vi "PH_Tektronix_7000.set Graph GUI Element.vi"(0 "i ref in":refnum<vi>, 5 "error in (no error)":errorcluster) -> (14 "i ref out":refnum<vi>, 19 "error out":errorcluster)   [LabVIEW 2014, in "PH_Tektronix_7000.lvlib"]
doc: "This sets the Graph GUI Element."
uses:
  PH_Tektronix_7000.lvlib
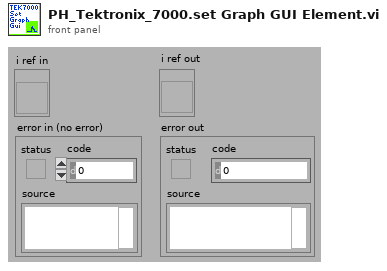
[diagram p1: front panel]
types:
  T1 = typedef "PH_Tektronix_7000.lvlib/PH_Tektronix_7000.i attribute.ctl" = cluster{"VISA Resource Name":refnum<visa-resource-name>, "IDN":cluster{"Instrument Driver":string, "Instrument Firmware":string, "Model":string, "Serial Number":string}, "Selftest":cluster{"Result":i32, "Message":string}, "Trigger Configuration":T2, "Acquisition Configuration":T3, "GUI Refs":T4, "State":T5, "Error Message":string, "Allow Prdc Loop?":bool, "Channel 1":T6, "Channel 2":T6, "Channel 3":T6, "Channel 4":T6, "Data CH 1":waveform(dbl), "Data CH 2":waveform(dbl), "Data CH 3":waveform(dbl), "Data CH 4":waveform(dbl), "Allow config?":bool, "Name Channel 1":string, "Name Channel 2":string, "Name Channel 3":string, "Name Channel 4":string, "Fetch Data before sending to PSDB?":bool, "Constructor passed?":bool, "Data taken at":timestamp, "Plot Colors":u32[], "Default VISA Resource":string}
  T2 = typedef "PH_Tektronix_7000.lvlib/PH_Tektronix_7000.Trigger Config.ctl" = cluster{"Source":u16, "Level [V]":dbl, "Slope":u16, "Coupling":u16, "Trigger Mode":u16}
  T3 = typedef "PH_Tektronix_7000.lvlib/PH_Tektronix_7000.Acquisition Config.ctl" = cluster{"Record Length":u32, "Timebase [s/div]":dbl, "Position [%]":dbl, "Acquisition Type":u16, "Average Waveforms":i32, "Envelope Waveforms":i32, "WfmDB Samples":i32, "Continuous?":bool, "Delay [s]":dbl, "Run?":bool}
  T4 = typedef "PH_Tektronix_7000.lvlib/PH_Tektronix_7000.GUI Refs.ctl" = cluster{"Graph":refnum<vi>, "State":refnum<vi>, "Delete":refnum<vi>, "VISA Resource":refnum<vi>, "Allow Configure":refnum<vi>, "Fetch Data":refnum<vi>, "Fetch before sending Data to PSDB":refnum<vi>, "Name Channel 1":refnum<vi>, "Name Channel 2":refnum<vi>, "Name Channel 3":refnum<vi>, "Name Channel 4":refnum<vi>, "Prdc Intervall [ms]":refnum<vi>, "Data taken":refnum<vi>, "Model":refnum<vi>, "Serial Number":refnum<vi>, "Firmware":refnum<vi>, "Driver":refnum<vi>, "Acquisition":refnum<vi>, "Trigger":refnum<vi>, "Cursor: D Time [s]":refnum<vi>, "Cursor: D Signal [V]":refnum<vi>, "Channel 1":refnum<vi>, "Channel 2":refnum<vi>, "Channel 3":refnum<vi>, "Channel 4":refnum<vi>}
  T5 = typedef "PH_StatusHandler.lvlib/PH_StatusHandler.Status.ctl" = i16
  T6 = typedef "PH_Tektronix_7000.lvlib/PH_Tektronix_7000.Channel Config.ctl" = cluster{"Enable Channel":bool, "Bandwidth":u16, "Input Impedance":u16, "Vertical Coupling":u16, "Probe Attenuation":dbl, "Range [V/div]":dbl, "Position [div]":dbl, "Bandwidth raw":string}
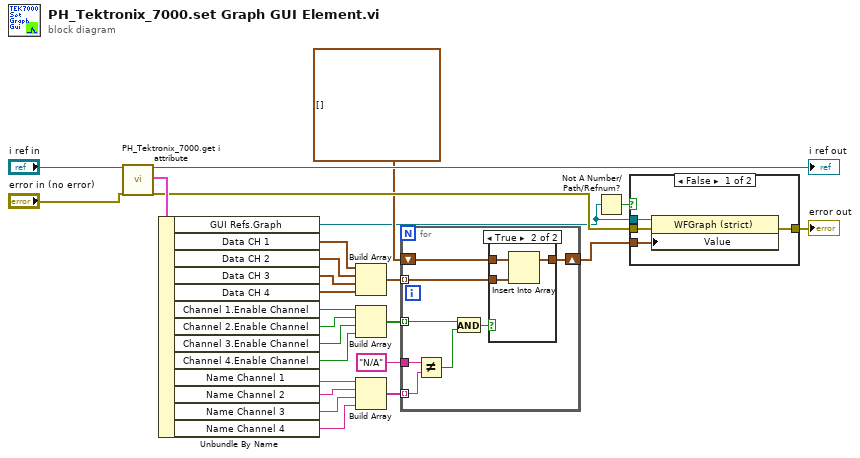
[diagram p0: block diagram]
diagram:
  n1 = call "PH_Tektronix_7000.get i attribute.vi"("i ref in"="i ref in", "error in (no error)"="error in (no error)") -> ("i ref out"=→"i ref out":refnum<vi>, "i attribute"=w26:T1, "error out"=w25:errorcluster)  [unwired: 15 in]
  n2 = Unbundle By Name(w26) -> ("GUI Refs.Graph"=w2:refnum<vi>, "Data CH 1"=w6:waveform(dbl), "Data CH 2"=w7:waveform(dbl), "Data CH 3"=w8:waveform(dbl), "Data CH 4"=w9:waveform(dbl), "Channel 1.Enable Channel"=w19:bool, "Channel 2.Enable Channel"=w18:bool, "Channel 3.Enable Channel"=w17:bool, "Channel 4.Enable Channel"=w16:bool, "Name Channel 1"=w15:string, "Name Channel 2"=w14:string, "Name Channel 3"=w13:string, "Name Channel 4"=w12:string)
  n3 = Build Array(w6, w7, w8, w9) -> (w5:waveform(dbl)[])
  n4 = Build Array(w19, w18, w17, w16) -> (w11:bool[])
  n5 = Build Array(w15, w14, w13, w12) -> (w10:string[])
  n6 = for {
    tunnel: w11 -> [w29] mode=indexing
    tunnel: w10 -> [w31] mode=indexing
    tunnel: w5 -> [w34] mode=indexing
    shift-right: [w33] -> w4
    shift-left: waveform(dbl)[] [] -> [w32]
    tunnel: "N/A" -> [w27]
    n7 = Not Equal?(x=w27, y=w31) -> (x != y?=w30:bool)
    n8 = And(x=w29, y=w30) -> (x .and. y?=w28:bool)
    n9 = case shown="True" w28 {
      tunnel: w34 -> [_ w38]
      tunnel: [w35 w37] -> w33
      tunnel: w32 -> [w35 w36]
      frame False {
      }
      frame True {
        n10 = Insert Into Array(array=w36, new element=w38) -> (w37:waveform(dbl)[])  [unwired: 1 in]
      }
    }
  }
  n11 = Not A Number/Path/Refnum?(number/path/refnum=w2) -> (NaN/Path/Refnum?=w21:bool)
  n12 = case shown="False" w21 {
    tunnel: w2 -> [w42 _]
    tunnel: w25 -> [w41 w43]
    tunnel: [w39 w43] -> w22
    tunnel: w4 -> [w40 _]
    frame False {
      n13 = property class="WFGraph (strict)"(reference=w42, error in=w41, "Value"=w40) -> (error out=w39:errorcluster)  [unwired: 1 out]
    }
    frame True {
    }
  }
  "error out" <- w22
